vi "Read UI Manipulation CMD.vi"(8 "error in (no error)":errorcluster, 11 "UI Console MSG in":refnum<class "UI Console MSG.lvclass">) -> (0 "error out":errorcluster, 2 "UI Manipulation CMD":i64, 3 "UI Console MSG out":refnum<class "UI Console MSG.lvclass">)   [LabVIEW 2024, in "UI Console MSG.lvclass"]
uses:
  UI Console MSG.lvclass
  UI Console MSG.lvclass/UI Console MSG.ctl
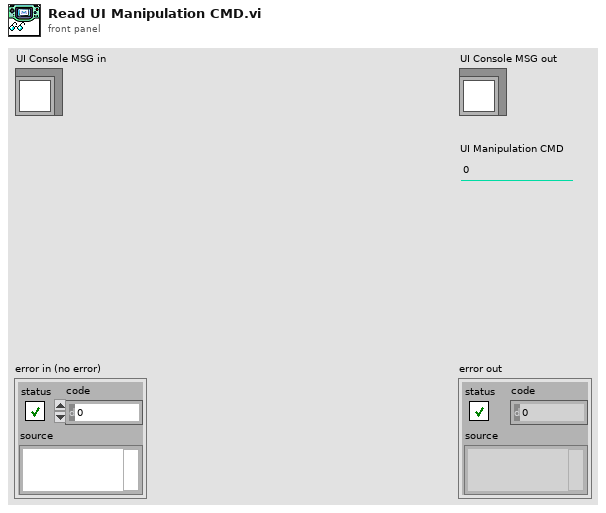
[diagram p1: front panel]
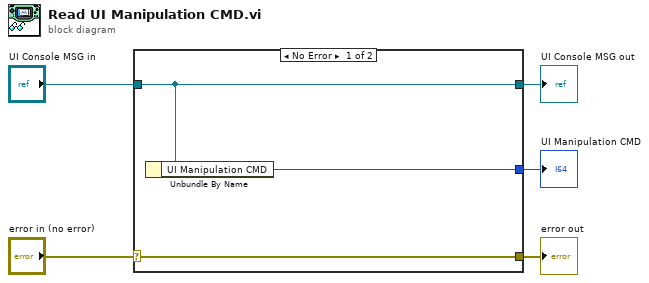
[diagram p0: block diagram]
diagram:
  n1 = case shown="No Error" "error in (no error)" {
    selector: "error in (no error)" -> [w8 w9]
    tunnel: [w8 w9] -> w4
    tunnel: [w7 w10] -> w2
    tunnel: "UI Console MSG in" -> [w7 w10]
    tunnel: [w6 _] -> w1
    frame No Error {
      n2 = Unbundle By Name(w7) -> ("UI Manipulation CMD"=w6:i64)
    }
    frame Error {
    }
  }
  "error out" <- w4
  "UI Console MSG out" <- w2
  "UI Manipulation CMD" <- w1
